vi "Print Panel.vi"(8 "error in (no error)":errorcluster, 9 "Entire Panel (T)":bool=TRUE, 11 "VI name":string) -> (0 "error out":errorcluster)   [LabVIEW 2016, in "generate report.lvlib"]
doc: "Produces the same printout as programmatic print at completion only if the front panel of the target VI is open before it runs."
uses:
  generate report.lvlib
panel:
  # "Entire"
  # "Visible"
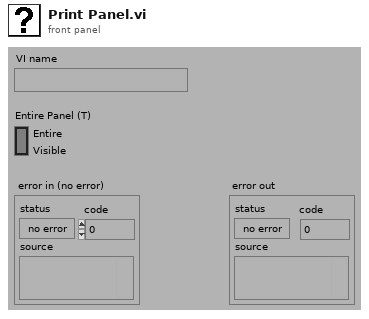
[diagram p1: front panel]
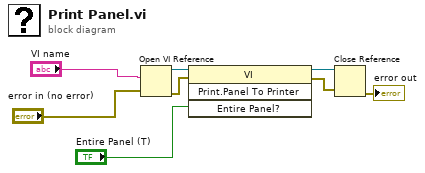
[diagram p0: block diagram]
diagram:
  n1 = Open VI Reference(vi path="VI name", error in (no error)="error in (no error)") -> (vi reference=w6:refnum<vi>, error out=w5:errorcluster)  [unwired: 4 in]
  n2 = invoke class="VI" method="Print.Panel To Printer"(reference=w6, error in=w5, "Entire Panel?"="Entire Panel (T)") -> (reference out=w3:refnum<vi>, error out=w2:errorcluster)  [unwired: 1 in, 2 out]
  n3 = Close Reference(reference=w3, error in (no error)=w2) -> (error out=→"error out":errorcluster)
